vi "Find Last Column Row.vi"(8 "error in":errorcluster, 11 "Excel._Worksheet":refnum<k7>) -> (0 "error out":errorcluster, 2 "Last column used:":u64, 3 "Last row used:":u64)   [LabVIEW 2017]
panel:
  out "ColumnWidth":variant
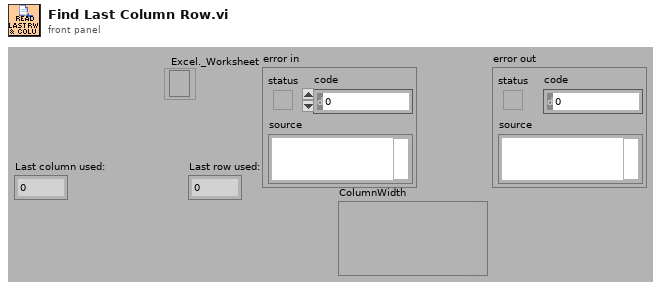
[diagram p1: front panel]
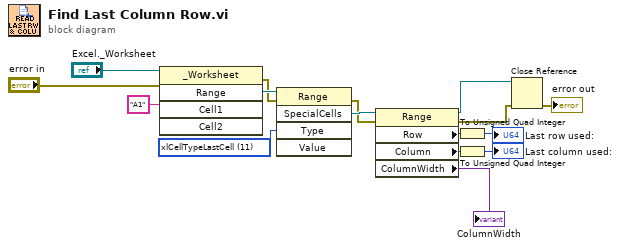
[diagram p0: block diagram]
diagram:
  w15 = 11 items=["xlCellTypeBlanks"=4, "xlCellTypeConstants"=2, "xlCellTypeFormulas"=-4123, "xlCellTypeLastCell"=11, "xlCellTypeComments"=-4144, "xlCellTypeVisible"=12, "xlCellTypeAllFormatConditions"=-4172, "xlCellTypeSameFormatConditions"=-4173, "xlCellTypeAllValidation"=-4174, "xlCellTypeSameValidation"=-4175] ("Type")
  n1 = invoke class="_Worksheet" method="Range"(reference="Excel._Worksheet", error in="error in", "Cell1"="A1") -> (error out=w9:errorcluster, "Range"=w13:refnum<k7>)  [unwired: 2 in, 3 out]
  n2 = invoke class="Range" method="SpecialCells"(reference=w13, error in=w9, "Type"=w15) -> (error out=w8:errorcluster, "SpecialCells"=w16:refnum<k7>)  [unwired: 2 in, 3 out]
  n3 = property class="Range"(reference=w16, error in=w8) -> (reference out=w7:refnum<k7>, error out=w6:errorcluster, "Row"=w14:i32, "Column"=w12:i32, "ColumnWidth"=→"ColumnWidth":variant)
  n4 = To Unsigned Quad Integer(1:w14) -> (0:→"Last row used:":u64)
  n5 = To Unsigned Quad Integer(1:w12) -> (0:→"Last column used:":u64)
  n6 = Close Reference(reference=w7, error in (no error)=w6) -> (error out=→"error out":errorcluster)
